vi "NI-DCPower LCR Advanced Sequence Voltage Sweep.vi"() -> ()   [LabVIEW 2020]
doc: "Overview: This example demonstrates how to make sweep times faster by using LCR Advanced Sequence functions to change the frequency in a sequence. During the sequence, the channel steps through the predetermined set configurations (frequency in this example) without any interaction with the host system. The advantage of sequencing is that changes from one step in the sequence to the next are deterministic.\nThe program will perform an AC Voltage frequency sweep from Start Frequency to End Frequency. The sweep frequencies are an exponential sequence and the length of each of the sweeps is equal to the value in the Number Of Steps control."
uses:
  <instrlib>/niDCPower/nidcpower.llb/niDCPower Source Mode.ctl
  <instrlib>/niDCPower/nidcpower.llb/niDCPower Wait For Event - Event.ctl
  <instrlib>/niDCPower/nidcpower.llb/niDCPower Sequence Attribute Type.ctl
  <instrlib>/niDCPower/nidcpower.llb/niDCPower Create Advanced Sequence Step With Channels.vi
  <vilib>/Utility/file.llb/Write Delimited Spreadsheet (DBL).vi
panel:
  in  "file path (use dialog)":path
  in  "Number of Steps":u32=100 caption="Number Of Steps"
  in  "Step Size":dbl=500000.0 format="%#_3p"
  in  "LCR Short Compensation Enabled":bool
  in  "LCR Open Compensation Enabled":bool
  in  "Impedance Range":dbl=100.0 format="%_6p"
  in  "Cable Length":i32(ring)=1123 items=["0m"=1121, "NI Standard 1m"=1122, "NI Standard 2m"=1123, "NI Standard 4m"=1124, "Custom (Onboard Storage)"=1125, "Custom (As Configured)"=1126, "NI Standard Triaxial 1m"=1139, "NI Standard Triaxial 2m"=1140, "NI Standard Triaxial 4m"=1141]
  in  "LCR Custom Measurement Time Sec":dbl caption="LCR Custom \nMeasurement Time Sec" format="%_3p"
  in  "LCR Measurement Time":i32(ring)=1072 items=["Short"=1071, "Medium"=1072, "Long"=1073, "Custom"=1117]
  in  "LCR DC Bias Source":i32(ring)=1066 items=["Off"=1065, "Voltage"=1066, "Current"=1067]
  in  "Voltage Amplitude RMS":dbl=0.7 format="%_6p"
  out "Impendance vs Frequency":T1(graph) caption="Impedance vs DC Voltage"
  in  "Channel Name":string="0"
  in  "Resource Name":refnum<k15>="Dev1"
  # "Overview: This example demonstrates how to make sweep times faster by using LCR Advanced Sequence functions to change the frequency in a sequence. During the sequence, the channel steps through the predetermined set configurations (frequency in this example) without any interaction with the host system. The advantage of sequencing is that changes from one step in the sequence to the next are deterministic. The program will perform an AC Voltage frequency sweep from Start Frequency to End Frequency. The sweep frequencies are an exponential sequence and the length of each of the sweeps is equal to the value in the Number Of Steps control. \n\nThe Cable Length option of \"Custom (As Configured)\" is not supported in this example. Search ni.com for information about NI power supplies/SMUs and the NI-DCPower API.\n\nRequirements: NI-DCPower\nInstructions:\n1. Select the appropriate instrument in the Resource Name control.\n2. Configure the parameters of the sweeps.\n3. Configure the Cable Length to match your cabling setup.\n4. Run the VI."
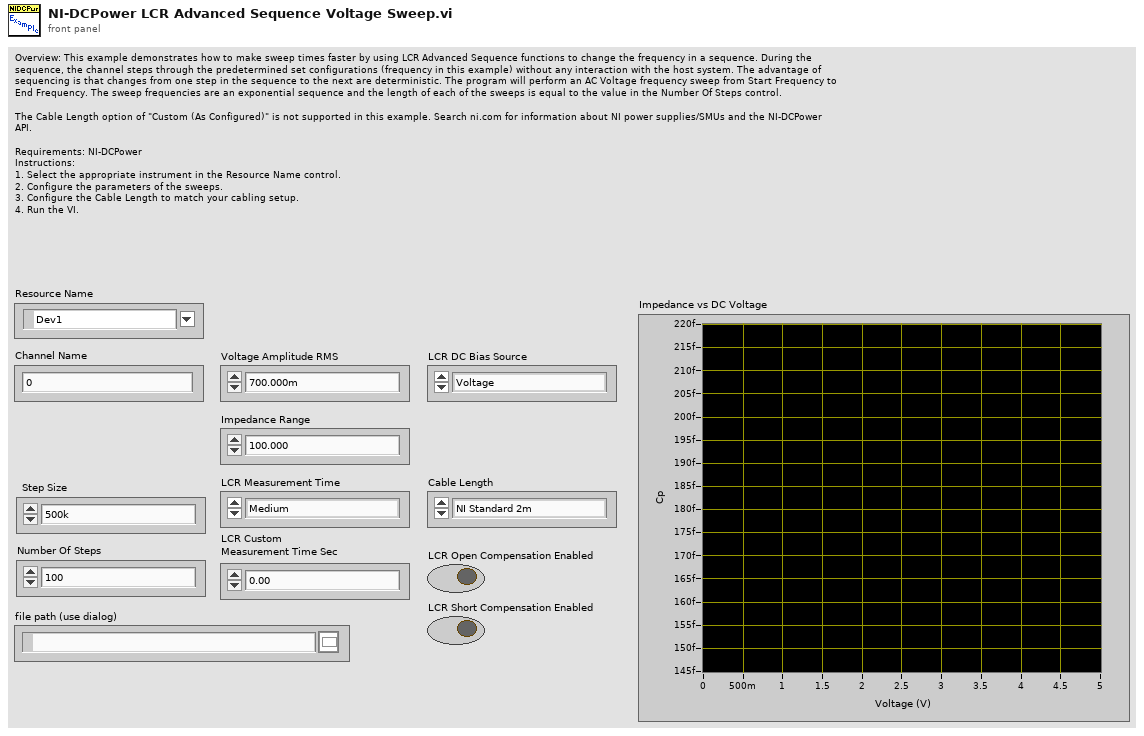
[diagram p1: front panel]
types:
  T1 = cluster{"voltage measurements":dbl[], "current measurements":dbl[]}
  T2 = typedef "niDCPower Sequence Attribute Type.ctl" = i32
  T3 = typedef "niDCPower Wait For Event - Event.ctl" = i32
  T4 = typedef "niDCPower Source Mode.ctl" = i32
  T5 = typedef "niDCPower LCR Measurement.ctl" = cluster{"V DC":dbl, "I DC":dbl, "stimulus frequency":dbl, "AC voltage":cdb, "AC current":cdb, "Z":cdb, "Z magnitude":dbl, "Z theta":dbl, "Y":cdb, "Y magnitude":dbl, "Y theta":dbl, "Ls":dbl, "Cs":dbl, "Rs":dbl, "Lp":dbl, "Cp":dbl, "Rp":dbl, "D":dbl, "Q":dbl, "measurement mode":u16, "DC in compliance":bool, "Pad 0":u8, "AC in compliance":bool, "Pad 1":u8, "unbalanced":bool, "Pad 2":u8, "Reserved 1":dbl, "Reserved 2":dbl, "Reserved 3":dbl, "Reserved 4":dbl, "Reserved 5":dbl, "Reserved 6":dbl, "Reserved 7":dbl}
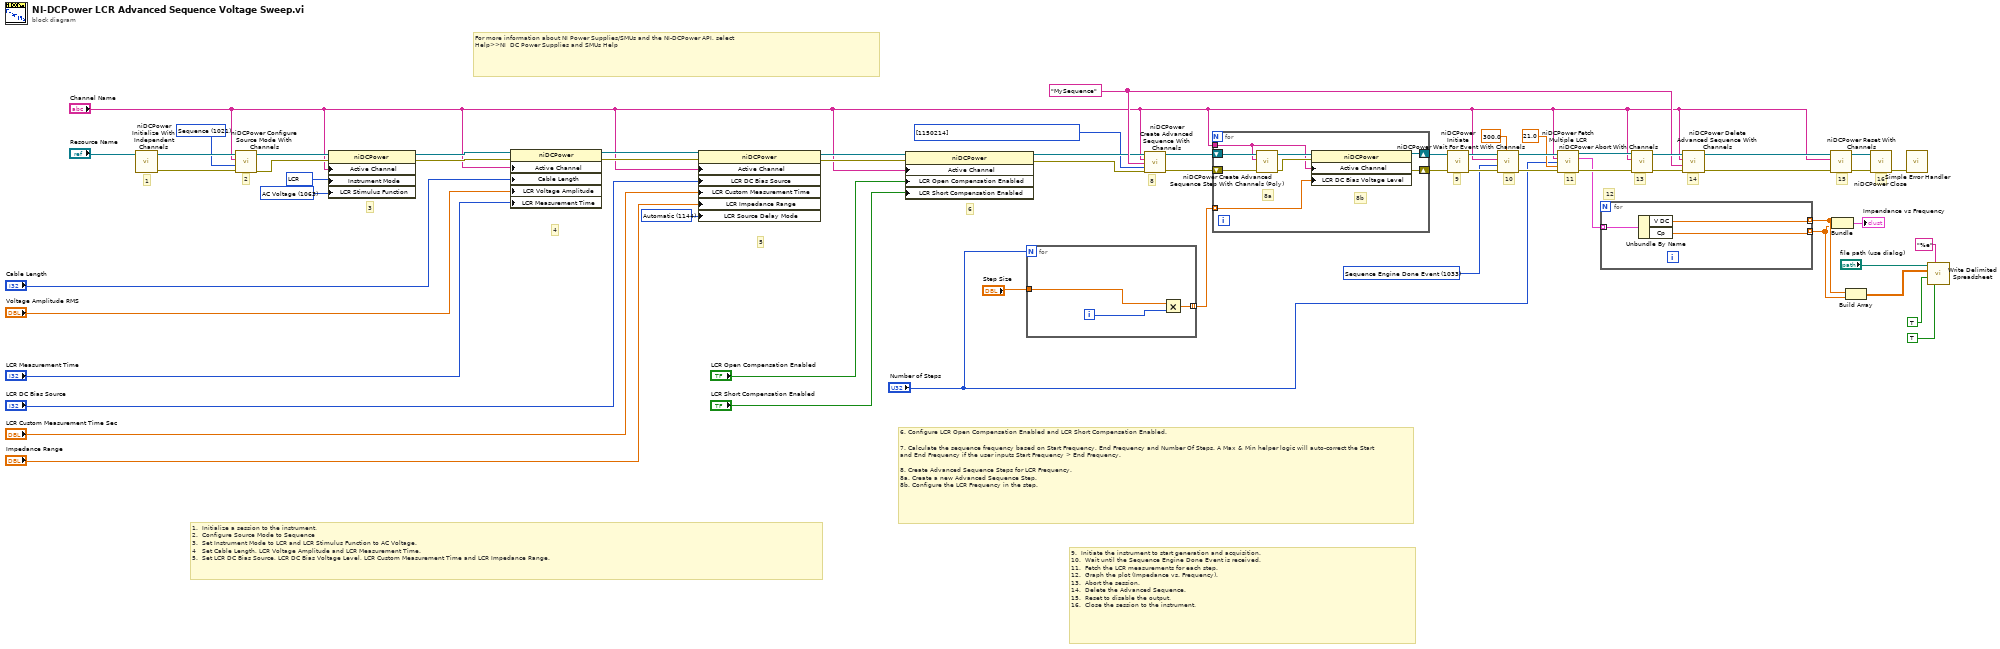
[diagram p0: block diagram]
diagram:
  w10 = 1144 items=["Automatic"=1144, "Manual"=1145] ("LCR:Source Delay Mode")
  w14 = T2[] [1150214] items=["Source -> Output Function"=1150008, "Source -> Output Enabled"=1250006, "Source -> Output Resistance"=1150061, "Source -> Transient Response"=1150062, "Source -> Custom Transient Response -> Voltage Gain Bandwidth"=1150067, "Source -> Custom Transient Response -> Voltage Compensation Frequency"=1150068, "Source -> Custom Transient Response -> Voltage Pole-Zero Ratio"=1150069, "Source -> Custom Transient Response -> Current Gain Bandwidth"=1150070, "Source -> Custom Transient Response -> Current Compensation Frequency"=1150071, "Source -> Custom Transient Response -> Current Pole-Zero Ratio"=1150072, "Source -> DC Voltage -> Voltage Level"=1250001, "Source -> DC Voltage -> Voltage Level Range"=1150005, "Source -> DC Voltage -> Current Limit"=1250005, "Source -> DC Voltage -> Current Limit High"=1150187, "Source -> DC Voltage -> Current Limit Low"=1150188, "Source -> DC Voltage -> Current Limit Range"=1150004, "Source -> DC Current -> Current Level"=1150009, "Source -> DC Current -> Current Level Range"=1150011, "Source -> DC Current -> Voltage Limit"=1150010, "Source -> DC Current -> Voltage Limit High"=1150185, "Source -> DC Current -> Voltage Limit Low"=1150186, "Source -> DC Current -> Voltage Limit Range"=1150012, "Source -> Pulse Voltage -> Pulse Voltage Level"=1150080, "Source -> Pulse Voltage -> Pulse Bias Voltage Level"=1150082, "Source -> Pulse Voltage -> Pulse Voltage Level Range"=1150084, "Source -> Pulse Voltage -> Pulse Current Limit"=1150081, "Source -> Pulse Voltage -> Pulse Current Limit High"=1150193, "Source -> Pulse Voltage -> Pulse Current Limit Low"=1150194, "Source -> Pulse Voltage -> Pulse Bias Current Limit"=1150083, "Source -> Pulse Voltage -> Pulse Bias Current Limit High"=1150195, "Source -> Pulse Voltage -> Pulse Bias Current Limit Low"=1150196, "Source -> Pulse Voltage -> Pulse Current Limit Range"=1150085, "Source -> Pulse Current -> Pulse Current Level"=1150086, "Source -> Pulse Current -> Pulse Bias Current Level"=1150088, "Source -> Pulse Current -> Pulse Current Level Range"=1150090, "Source -> Pulse Current -> Pulse Voltage Limit"=1150087, "Source -> Pulse Current -> Pulse Voltage Limit High"=1150189, "Source -> Pulse Current -> Pulse Voltage Limit Low"=1150190, "Source -> Pulse Current -> Pulse Bias Voltage Limit"=1150089, "Source -> Pulse Current -> Pulse Bias Voltage Limit High"=1150191, "Source -> Pulse Current -> Pulse Bias Voltage Limit Low"=1150192, "Source -> Pulse Current -> Pulse Voltage Limit Range"=1150091, "Source -> Advanced -> Source Delay"=1150051, "Source -> Advanced -> Pulse Bias Delay"=1150092, "Source -> Advanced -> Pulse On Time"=1150093, "Source -> Advanced -> Pulse Off Time"=1150094, "Source -> Advanced -> OVP Enabled"=1250002, "Source -> Advanced -> OVP Limit"=1250003, "Source -> Advanced -> Compliance Limit Symmetry"=1150184, "Source -> Advanced -> Sequence Step Delta Time"=1150198, "Measurement -> Sense"=1150013, "Measurement -> Aperture Time"=1150058, "Measurement -> Measure Record Length"=1150063, "Measurement -> Advanced -> DC Noise Rejection"=1150066, "Measurement -> Autorange"=1150244, "Measurement -> Advanced -> Autorange Behavior"=1150245, "Measurement -> Advanced -> Autorange Aperture Time Mode"=1150246, "Measurement -> Advanced -> Autorange Minimum Aperture Time"=1150247, "Measurement -> Advanced -> Autorange Minimum Aperture Time Units"=1150248, "Measurement -> Advanced -> Autorange Minimum Current Range"=1150255, "Measurement -> Advanced -> Autorange Minimum Voltage Range"=1150256, "Measurement -> Advanced -> Autorange Threshold Mode"=1150257, "Measurement -> Advanced -> Autorange Maximum Delay After Range Change"=1150322, "LCR -> Instrument Mode"=1150208, "LCR -> Source Delay Mode"=1150315, "LCR -> Measurement Time"=1150218, "LCR -> Custom Measurement Time"=1150258, "LCR -> AC Stimulus -> Function"=1150209, "LCR -> AC Stimulus -> Frequency"=1150210, "LCR -> AC Stimulus -> Voltage Amplitude"=1150211, "LCR -> AC Stimulus -> Current Amplitude"=1150212, "LCR -> AC Stimulus -> Advanced -> Voltage Range"=1150265, "LCR -> AC Stimulus -> Advanced -> Current Range"=1150267, "LCR -> DC Bias -> Source"=1150213, "LCR -> DC Bias -> Voltage Level"=1150214, "LCR -> DC Bias -> Current Level"=1150215, "LCR -> DC Bias -> Advanced -> Voltage Range"=1150266, "LCR -> DC Bias -> Advanced -> Current Range"=1150274, "LCR -> Compensation -> Open -> Enabled"=1150220, "LCR -> Compensation -> Open -> Conductance"=1150261, "LCR -> Compensation -> Open -> Susceptance"=1150262, "LCR -> Compensation -> Short -> Enabled"=1150221, "LCR -> Compensation -> Short -> Resistance"=1150263, "LCR -> Compensation -> Short -> Reactance"=1150264, "LCR -> Compensation -> Load -> Enabled"=1150222, "LCR -> Compensation -> Load -> Measured Resistance"=1150268, "LCR -> Compensation -> Load -> Measured Reactance"=1150269, "LCR -> Compensation -> Load -> Actual Resistance"=1150270, "LCR -> Compensation -> Load -> Actual Reactance"=1150271, "LCR -> Impedance Range -> Impedance Range"=1150217, "LCR -> Impedance Range -> Impedance Autorange"=1150216, "LCR -> Impedance Range -> Advanced -> Impedance Range Source"=1150321, "LCR -> Impedance Range -> Advanced -> Load Resistance"=1150318, "LCR -> Impedance Range -> Advanced -> Load Inductance"=1150319, "LCR -> Impedance Range -> Advanced -> Load Capacitance"=1150320] ("advanced sequence properties")
  w33 = 1063 items=["AC Voltage"=1063, "AC Current"=1064] ("LCR:AC Stimulus:Function")
  w36 = 1062 items=["SMU PS"=1061, "LCR"=1062] ("LCR:Instrument Mode")
  w39 = "MySequence" ("sequence name")
  w50 = T3 1033 items=["Source Complete Event"=1030, "Measure Complete Event"=1031, "Sequence Iteration Complete Event"=1032, "Sequence Engine Done Event"=1033] ("event")
  w55 = T4 1021 items=["Single Point"=1020, "Sequence"=1021] ("source mode")
  # "1"
  # "5"
  # "6. Configure LCR Open Compensation Enabled and LCR Short Compensation Enabled.\n\n7. Calculate the sequence frequency based on Start Frequency, End Frequency and Number Of Steps. A Max & Min helper logic will auto-correct the Start and End Frequency if the user inputs Start Frequency > End Frequency.\n\n8. Create Advanced Sequence Steps for LCR Frequency.\n8a. Create a new Advanced Sequence Step.\n8b. Configure the LCR Frequency in the step."
  # "6"
  # "4"
  # "3"
  # "8"
  # "13"
  # "14"
  # "9.  Initiate the instrument to start generation and acquisition.\n10.  Wait until the Sequence Engine Done Event is received.\n11.  Fetch the LCR measurements for each step.\n12.  Graph the plot (Impedance vs. Frequency).\n13.  Abort the session.\n14.  Delete the Advanced Sequence.\n15.  Reset to disable the output.\n16.  Close the session to the instrument."
  # "For more information about NI Power Supplies/SMUs and the NI-DCPower API, select\nHelp>>NI  DC Power Supplies and SMUs Help"
  # "16"
  # "9"
  # "11"
  # "10"
  # "2"
  # "1.  Initialize a session to the instrument.\n2.  Configure Source Mode to Sequence \n3.  Set Instrument Mode to LCR and LCR Stimulus Function to AC Voltage.\n4   Set Cable Length, LCR Voltage Amplitude and LCR Measurement Time. \n5.  Set LCR DC Bias Source, LCR DC Bias Voltage Level, LCR Custom Measurement Time and LCR Impedance Range."
  # "12"
  # "15"
  n1 = call <instrlib>:"niDCPower Initialize With Independent Channels.vi"("resource name"="Resource Name") -> ("error out"=w57:errorcluster, "instrument handle out"=w56:refnum<k15>)  [unwired: 9 in]
  n2 = call <instrlib>:"niDCPower Configure Source Mode With Channels.vi"("error in (no error)"=w57, "source mode"=w55, "channel name"="Channel Name", "instrument handle"=w56) -> ("error out"=w42:errorcluster, "instrument handle out"=w43:refnum<k15>)  [unwired: 6 in]
  n3 = property class="niDCPower"(reference=w43, error in=w42, "Active Channel"="Channel Name", "Instrument Mode"=w36, "LCR Stimulus Function"=w33) -> (reference out=w25:refnum<k15>, error out=w24:errorcluster)
  n4 = property class="niDCPower"(reference=w25, error in=w24, "Active Channel"="Channel Name", "Cable Length"="Cable Length", "LCR Voltage Amplitude"="Voltage Amplitude RMS", "LCR Measurement Time"="LCR Measurement Time") -> (reference out=w23:refnum<k15>, error out=w22:errorcluster)
  n5 = property class="niDCPower"(reference=w23, error in=w22, "Active Channel"="Channel Name", "LCR DC Bias Source"="LCR DC Bias Source", "LCR Custom Measurement Time"="LCR Custom Measurement Time Sec", "LCR Impedance Range"="Impedance Range", "LCR Source Delay Mode"=w10) -> (reference out=w31:refnum<k15>, error out=w30:errorcluster)
  n6 = property class="niDCPower"(reference=w31, error in=w30, "Active Channel"="Channel Name", "LCR Open Compensation Enabled"="LCR Open Compensation Enabled", "LCR Short Compensation Enabled"="LCR Short Compensation Enabled") -> (reference out=w29:refnum<k15>, error out=w28:errorcluster)
  n7 = for {
    N: "Number of Steps" -> [_]
    tunnel: [w63] -> w13 mode=indexing
    tunnel: "Step Size" -> [w62]
    i -> [w61]
    n8 = Multiply(x=w62, y=w61) -> (x*y=w63:dbl)
  }
  n9 = call <instrlib>:"niDCPower Create Advanced Sequence With Channels.vi"("instrument handle"=w29, "channel name"="Channel Name", "sequence name"=w39, "advanced sequence properties"=w14, "error in (no error)"=w28) -> ("instrument handle out"=w41:refnum<k15>, "error out"=w40:errorcluster)  [unwired: 9 in]
  n10 = for {
    shift-right: [w68] -> w37
    shift-left: w40 -> [w71]
    tunnel: w13 -> [w65] mode=indexing
    tunnel: "Channel Name" -> [w64]
    shift-right: [w66] -> w38
    shift-left: w41 -> [w70]
    # "8b"
    # "8a"
    n11 = call-poly <instrlib>:"niDCPower Create Advanced Sequence Step With Channels (Poly).vi"("error in (no error)"=w71, "channel name"=w64, "instrument handle"=w70) -> ("error out"=w67:errorcluster, "instrument handle out"=w69:refnum<k15>)  [unwired: 7 in]
    n12 = property class="niDCPower"(reference=w69, error in=w67, "Active Channel"=w64, "LCR DC Bias Voltage Level"=w65) -> (reference out=w66:refnum<k15>, error out=w68:errorcluster)
  }
  n13 = call <instrlib>:"niDCPower Initiate.vi"("error in (no error)"=w37, "instrument handle"=w38) -> ("error out"=w52:errorcluster, "instrument handle out"=w54:refnum<k15>)  [unwired: 2 in, 6 out]
  n14 = call <instrlib>:"niDCPower Wait For Event With Channels.vi"("timeout (10.0)"=300.0, "error in (no error)"=w52, "event"=w50, "channel name"="Channel Name", "instrument handle"=w54) -> ("error out"=w51:errorcluster, "instrument handle out"=w53:refnum<k15>)  [unwired: 5 in]
  n15 = call <instrlib>:"niDCPower Fetch Multiple LCR.vi"("instrument handle"=w53, "channel name"="Channel Name", "count (1)"="Number of Steps", "timeout (1.0)"=21.0, "error in (no error)"=w51) -> ("instrument handle out"=w45:refnum<k15>, "measurements"=w35:T5[], "error out"=w47:errorcluster)  [unwired: 7 in, 1 out]
  n16 = for {
    tunnel: w35 -> [w74] mode=indexing
    tunnel: [w73] -> w8 mode=indexing
    tunnel: [w72] -> w7 mode=indexing
    n17 = Unbundle By Name(w74) -> ("V DC"=w73:dbl, "Cp"=w72:dbl)
  }
  n18 = call <instrlib>:"niDCPower Abort With Channels.vi"("error in (no error)"=w47, "channel name"="Channel Name", "instrument handle"=w45) -> ("error out"=w46:errorcluster, "instrument handle out"=w44:refnum<k15>)  [unwired: 7 in]
  n19 = call <instrlib>:"niDCPower Delete Advanced Sequence With Channels.vi"("error in (no error)"=w46, "sequence name"=w39, "channel name"="Channel Name", "instrument handle"=w44) -> ("error out"=w49:errorcluster, "instrument handle out"=w48:refnum<k15>)  [unwired: 6 in]
  n20 = call <instrlib>:"niDCPower Reset With Channels.vi"("error in (no error)"=w49, "channel name"="Channel Name", "instrument handle"=w48) -> ("error out"=w59:errorcluster, "instrument handle out"=w60:refnum<k15>)  [unwired: 7 in]
  n21 = Bundle(w8, w7) -> (→"Impendance vs Frequency":cluster{dbl[], dbl[]})  [unwired: 1 out]
  n22 = Build Array(w8, w7) -> (w6:dbl[][])
  n23 = call <instrlib>:"niDCPower Close.vi"("error in (no error)"=w59, "instrument handle"=w60) -> ("error out"=w58:errorcluster)  [unwired: 9 out]
  n24 = call <vilib>:"Simple Error Handler.vi"("error in (no error)"=w58) -> ()  [unwired: 1 in, 8 out]
  n25 = call-poly <vilib>:"Write Delimited Spreadsheet.vi"("file path (dialog if empty)"="file path (use dialog)", "format (%.3f)"="%e", "2D data"=w6, "append to file? (new file:F)"=TRUE, "transpose? (no:F)"=TRUE) -> ()  [unwired: 9 in, 2 out]
